vi "PQgetCopyData.vi"(8 "error in (no error)":errorcluster, 9 "async":i32, 10 "buffer":u32, 11 "conn":u32) -> (0 "error out":errorcluster, 1 "PQgetCopyData":i32, 2 "buffer_out":u32, 3 "conn_out":u32)   [LabVIEW 2019, in "libpqlv.lvlib"]
uses:
  libpqlv.lvlib
  libpq.dll
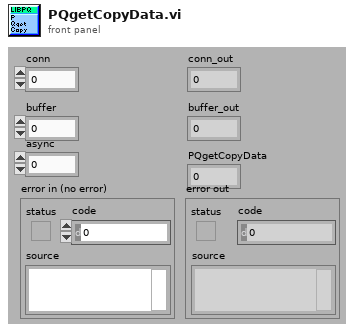
[diagram p1: front panel]
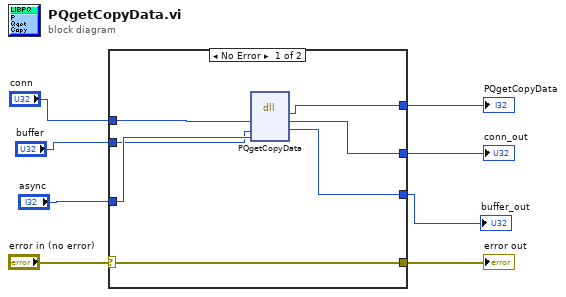
[diagram p0: block diagram]
diagram:
  n1 = case shown="No Error" "error in (no error)" {
    selector: "error in (no error)" -> [w15 w18]
    tunnel: [w15 w18] -> w7
    tunnel: [w14 _] -> w6
    tunnel: [w13 w17] -> w5
    tunnel: "async" -> [w12 _]
    tunnel: "conn" -> [w11 w17]
    tunnel: [w10 w16] -> w1
    tunnel: "buffer" -> [w9 w16]
    frame No Error {
      n2 = dll-call lib="libpq.*" fn="PQgetCopyData"("conn"=w11, "buffer"=w9, "async"=w12) -> ("PQgetCopyData"=w14:i32, "conn"=w13:u32, "buffer"=w10:u32)  [unwired: 4 in, 2 out]
    }
    frame Error {
    }
  }
  "PQgetCopyData" <- w6
  "error out" <- w7
  "conn_out" <- w5
  "buffer_out" <- w1
